vi "RobotDLLToolInit (SubVI).vi"(4 "Target Tool Withdraw Speed":dbl, 5 "Target Tool Insertion Speed":dbl, 6 "Target Tool Withdraw Length":dbl, 7 "Target Tool Insertion Length":dbl, 8 "Tool Fast Retraction":bool, 9 "Tool Withdraw":bool, 10 "Tool Insertion":bool, 11 "ArmID":i32) -> (0 "actInsertionLength":dbl)   [LabVIEW 2016]
uses:
  EyeRobotDLL.dll
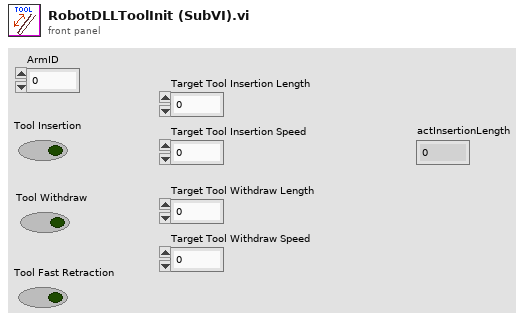
[diagram p1: front panel]
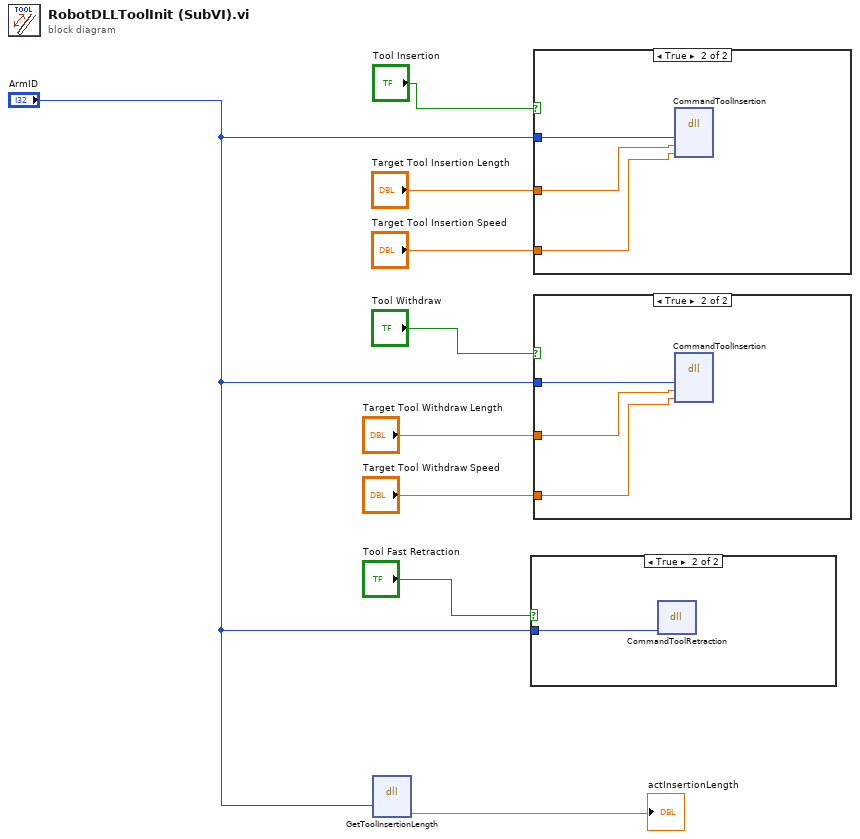
[diagram p0: block diagram]
diagram:
  n1 = dll-call lib="D:/IRISSoft LV2016 beta/Host Demo Subsystems/EyeRobotDLL.dll" fn="GetToolInsertionLength"("id"="ArmID") -> ("insertionLength"=→"actInsertionLength":dbl)  [unwired: 6 in, 2 out]
  n2 = case shown="True" "Tool Fast Retraction" {
    tunnel: "ArmID" -> [_ w10]
    frame False {
    }
    frame True {
      n3 = dll-call lib="D:/IRISSoft LV2016 beta/Host Demo Subsystems/EyeRobotDLL.dll" fn="CommandToolRetraction"("id"=w10) -> ()  [unwired: 5 in, 2 out]
    }
  }
  n4 = case shown="True" "Tool Insertion" {
    tunnel: "ArmID" -> [_ w13]
    tunnel: "Target Tool Insertion Length" -> [_ w12]
    tunnel: "Target Tool Insertion Speed" -> [_ w11]
    frame False {
    }
    frame True {
      n5 = dll-call lib="D:/IRISSoft LV2016 beta/Host Demo Subsystems/EyeRobotDLL.dll" fn="CommandToolInsertion"("id"=w13, "insertionLength"=w12, "speed"=w11) -> ()  [unwired: 7 in, 2 out]
    }
  }
  n6 = case shown="True" "Tool Withdraw" {
    tunnel: "ArmID" -> [_ w16]
    tunnel: "Target Tool Withdraw Length" -> [_ w15]
    tunnel: "Target Tool Withdraw Speed" -> [_ w14]
    frame False {
    }
    frame True {
      n7 = dll-call lib="D:/IRISSoft LV2016 beta/Host Demo Subsystems/EyeRobotDLL.dll" fn="CommandToolInsertion"("id"=w16, "insertionLength"=w15, "speed"=w14) -> ()  [unwired: 7 in, 2 out]
    }
  }
